vi "VeriStand DSF.Transfer Group.Configuration.Verify.Channels Configuration.vi"(8 "error in (no error)":errorcluster, 11 "Transfer Group Configuration in":refnum<class "VeriStand DSF.Transfer Group.Configuration.lvclass">=refnum) -> (0 "error out":errorcluster, 3 "Transfer Group Configuration out":refnum<class "VeriStand DSF.Transfer Group.Configuration.lvclass">)   [LabVIEW 2017, in "Data Sharing Custom Device Engine.lvlib" / "VeriStand DSF.Transfer Group.Configuration.lvclass"]
uses:
  VeriStand DSF.Transfer Group.Configuration.lvclass
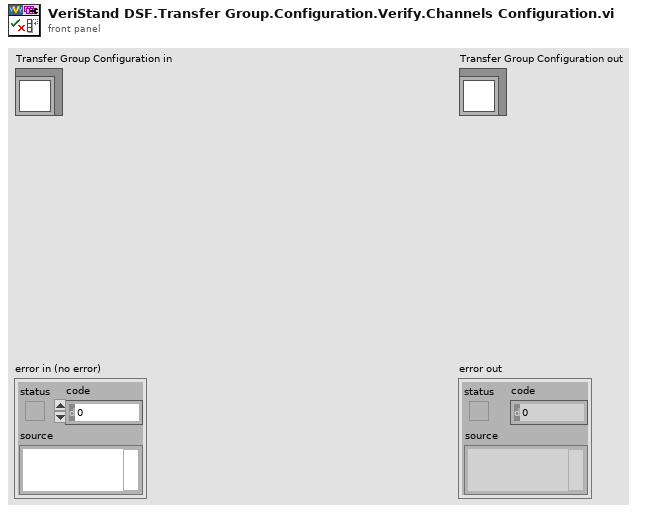
[diagram p1: front panel]
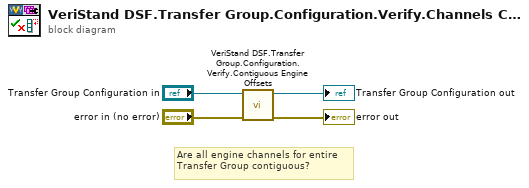
[diagram p0: block diagram]
diagram:
  # "Are all engine channels for entire Transfer Group contiguous?"
  n1 = call "VeriStand DSF.Transfer Group.Configuration.Verify.Contiguous Engine Offsets.vi"("error in (no error)"="error in (no error)", "Transfer Group Configuration in"="Transfer Group Configuration in") -> ("error out"=→"error out":errorcluster, "Transfer Group Configuration out"=→"Transfer Group Configuration out":refnum<class "VeriStand DSF.Transfer Group.Configuration.lvclass">)  [unwired: 8 in]
